vi "cm2nm_Init_table_on_sampleInfo.vi"(2 "Sample_Information":T2, 3 "Sample locations of Interest":refnum<vi>, 4 "TopLevelDataFilePath":path) -> ()   [LabVIEW 2011]
doc: "Populate the table from sample information. This will read the session files and create a list of the sample locations and set indications for what sessions particular sample locations have be included."
uses:
  cm2nm_coordinate_information_v2.ctl
panel:
  out "CollectionOfPoints":T1[](array[typedef])
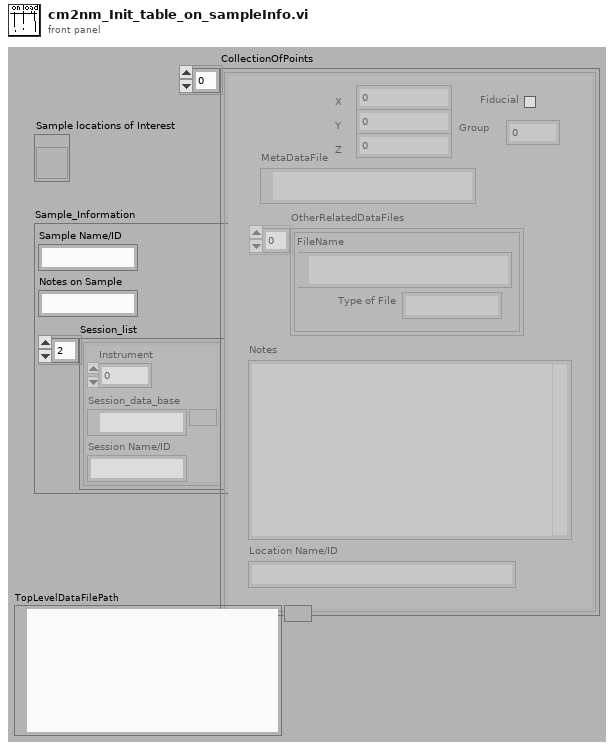
[diagram p1: front panel]
types:
  T1 = typedef "cm2nm_coordinate_information_v2.ctl" = cluster{"MetaDataFile":path, "X":dbl, "Y":dbl, "Z":dbl, "Group":i32, "Rotation":dbl[unit], "Fiducial":bool, "Magnification":dbl, "Working_Distance":dbl, "Notes":string, "Location Name/ID":string, "OtherRelatedDataFiles":cluster{"Type of File":string, "FileName":path}[], "Available":bool}
  T2 = cluster{"Sample Name/ID":string, "Notes on Sample":string, "Session_list":cluster{"Instrument":u16, "Session_data_base":path, "Session Name/ID":string}[]}
  T3 = cluster{"Instrument":u16, "Session_data_base":path, "Session Name/ID":string}[]
  T4 = typedef "cm2nm_sample_set.ctl" = cluster{"CollectionOfPoints":T1[], "Instrument":T5, "CollectionFile":path, "Session Name/ID":string, "SessionNotes":string}
  T5 = typedef "Instrument_type_enum_v2.ctl" = enum16{"Unknown", "Philips FEI SEM IRC", "JEOL 7000F EML_MFC", "MXRD MFC", "JEOL_EPMA"}
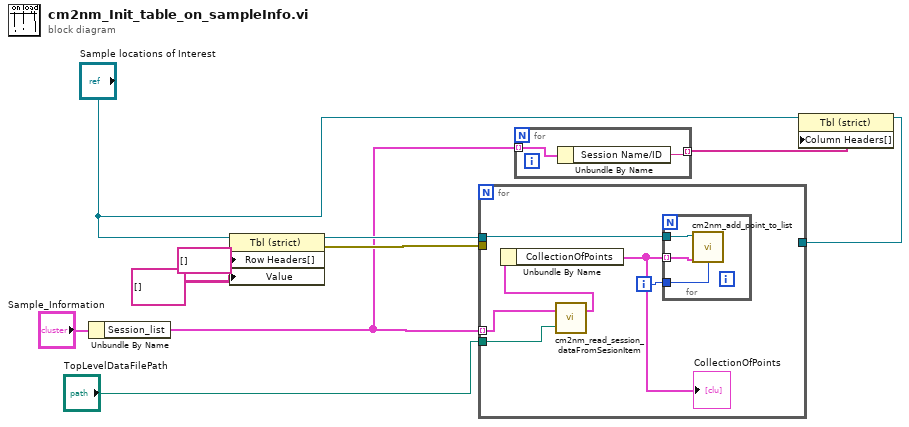
[diagram p0: block diagram]
diagram:
  n1 = Unbundle By Name("Sample_Information") -> ("Session_list"=w3:T3)
  n2 = property on="Property Node" class="Tbl (strict)"(reference="Sample locations of Interest", "Row Headers[]"=string[] [] ("Row Header Strings[]"), "Value"=string[][] [] ("Sample locations of Interest")) -> (reference out=w8:refnum<vi>, error out=w7:errorcluster)  [unwired: 1 in]
  n3 = for {
    tunnel: w3 -> [w12] mode=indexing
    tunnel: [w11] -> w2 mode=indexing
    n4 = Unbundle By Name(w12) -> ("Session Name/ID"=w11:string)
  }
  n5 = property on="Property Node" class="Tbl (strict)"(reference="Sample locations of Interest", "Column Headers[]"=w2) -> (reference out=w1:refnum<vi>)  [unwired: 1 in, 1 out]
  n6 = for {
    tunnel: w3 -> [w17] mode=indexing
    tunnel: w7 -> [_]
    tunnel: w8 -> [w14]
    tunnel: "TopLevelDataFilePath" -> [w13]
    tunnel: w1 -> [_]
    i -> [w15]
    n7 = call "cm2nm_read_session_dataFromSesionItem.vi"("TopLevelDataFilePath"=w13, "Sesions"=w17) -> ("Session_OUT"=w18:T4)  [unwired: 1 in]
    n8 = Unbundle By Name(w18) -> ("CollectionOfPoints"=w16:T1[])
    "CollectionOfPoints" <- w16
    n9 = for {
      tunnel: w16 -> [w21] mode=indexing
      tunnel: w15 -> [w20]
      tunnel: w14 -> [w19]
      n10 = call "cm2nm_add_point_to_list.vi"("SampleDataPoint"=w21, "SessionIndex"=w20, "Sample locations of Interest"=w19) -> ()  [unwired: 1 out]
    }
  }
